vi "Build dotNET Product List.vi"(8 "error in (no error)":errorcluster, 11 "Bundle Builder in":refnum<class "Bundle Builder.lvclass">) -> (0 "error out":errorcluster, 2 "Product List":refnum<k24>[](array[refnum]), 3 "Bundle Builder out":refnum<class "Bundle Builder.lvclass">)   [LabVIEW 2020, in "Bundle Builder.lvclass"]
uses:
  Bundle Builder.lvclass
  C:/Users/chihong/Documents/Repos/StsCustomBundleBuilder/Code/StsCustomBundleBuilder/StsCustomBundleBuilderLib/StsCustomBundleBuilderLib.dll
  StsCustomBundleBuilderLib/StsCustomBundleBuilderLib.dll
  Bundle Builder.lvclass/Bundle Builder.ctl
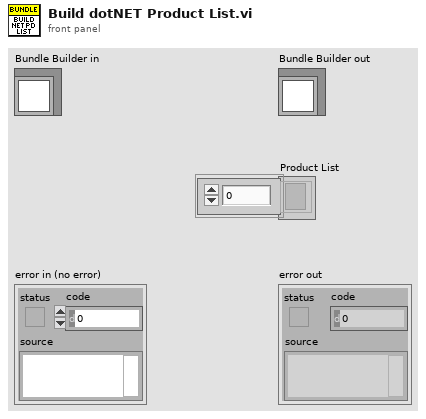
[diagram p1: front panel]
types:
  T1 = cluster{"Display Name":string, "Type":enum16{"NI Installer", "Custom Installer"}, "Install Commands":cluster{"Path":string, "Parameters":string, "Successful Exit Codes":string, "Log Command":cluster{"Flag":string, "File Name":string}}[], "Uninstall Commands":cluster{"Path":string, "Parameters":string, "Successful Exit Codes":string, "Log Command":cluster{"Flag":string, "File Name":string}}[]}[]
  T2 = cluster{"Path":string, "Parameters":string, "Successful Exit Codes":string, "Log Command":cluster{"Flag":string, "File Name":string}}[]
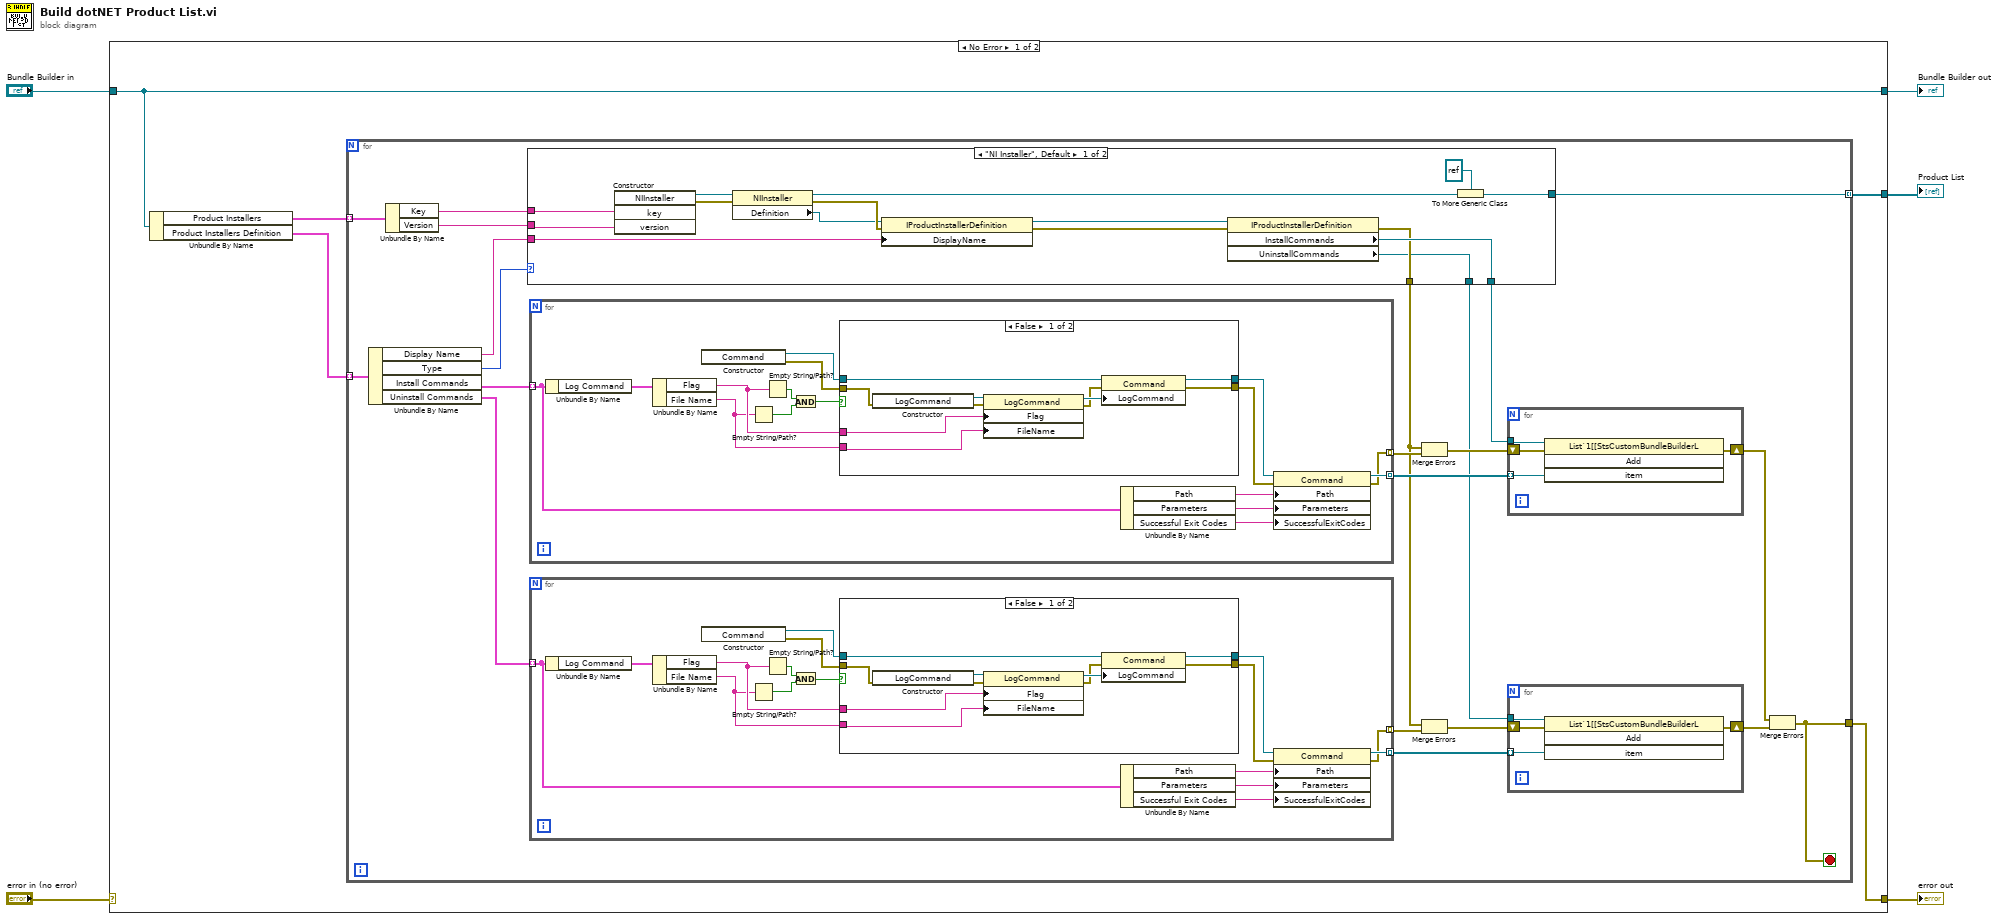
[diagram p0: block diagram]
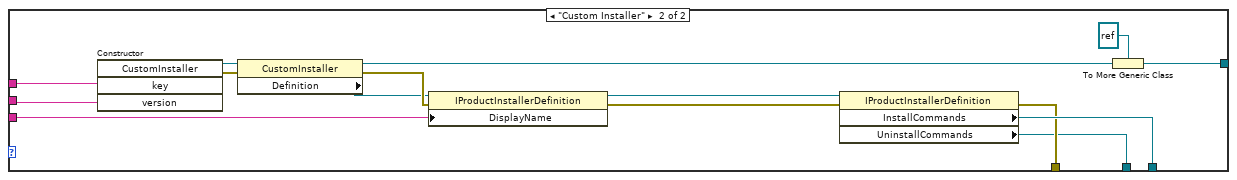
[diagram p3: hidden frame]
diagram:
  n1 = case shown="No Error" "error in (no error)" {
    selector: "error in (no error)" -> [_ w127]
    tunnel: [w7 w127] -> w4
    tunnel: [w8 w126] -> w2
    tunnel: "Bundle Builder in" -> [w8 w126]
    tunnel: [w6 _] -> w1
    frame No Error {
      n2 = Unbundle By Name(w8) -> ("Product Installers"=w10:cluster{"Key":string, "Version":string}[], "Product Installers Definition"=w9:T1)
      n3 = for {
        tunnel: w10 -> [w28] mode=indexing
        tunnel: w9 -> [w31] mode=indexing
        tunnel: [w12] -> w7
        tunnel: [w11] -> w6 mode=indexing
        stop <- w12 stop-if-true
        n4 = Unbundle By Name(w31) -> ("Display Name"=w27:string, "Type"=w29:enum16{"NI Installer", "Custom Installer"}, "Install Commands"=w30:T2, "Uninstall Commands"=w17:T2)
        n5 = Unbundle By Name(w28) -> ("Key"=w25:string, "Version"=w26:string)
        n6 = case shown="\"NI Installer\", Default" w29 {
          tunnel: w27 -> [w81 w96]
          tunnel: w26 -> [w74 w89]
          tunnel: w25 -> [w75 w90]
          tunnel: [w79 w94] -> w24
          tunnel: [w77 w92] -> w16
          tunnel: [w76 w91] -> w15
          tunnel: [w68 w83] -> w11
          frame "NI Installer", Default {
            n7 = constructor class="NIInstaller"("key"=w75, "version"=w74) -> (reference out=w72:refnum<k24>, error out=w82:errorcluster)  [unwired: 3 in, 3 out]
            n8 = property class="NIInstaller"(reference=w72, error in=w82) -> (reference out=w69:refnum<k24>, error out=w73:errorcluster, "Definition"=w71:refnum<k24>)
            n9 = property class="IProductInstallerDefinition"(reference=w71, error in=w73, "DisplayName"=w81) -> (reference out=w80:refnum<k24>, error out=w78:errorcluster)
            n10 = property class="IProductInstallerDefinition"(reference=w80, error in=w78) -> (error out=w77:errorcluster, "InstallCommands"=w79:refnum<k24>, "UninstallCommands"=w76:refnum<k24>)  [unwired: 1 out]
            n11 = To More Generic Class(target class=refnum<k24> refnum ("new reference"), reference=w69) -> (generic class reference=w68:refnum<k24>)
          }
          frame "Custom Installer" {
            n12 = constructor class="CustomInstaller"("key"=w90, "version"=w89) -> (reference out=w87:refnum<k24>, error out=w97:errorcluster)  [unwired: 3 in, 3 out]
            n13 = property class="CustomInstaller"(reference=w87, error in=w97) -> (reference out=w84:refnum<k24>, error out=w88:errorcluster, "Definition"=w86:refnum<k24>)
            n14 = property class="IProductInstallerDefinition"(reference=w86, error in=w88, "DisplayName"=w96) -> (reference out=w95:refnum<k24>, error out=w93:errorcluster)
            n15 = property class="IProductInstallerDefinition"(reference=w95, error in=w93) -> (error out=w92:errorcluster, "InstallCommands"=w94:refnum<k24>, "UninstallCommands"=w91:refnum<k24>)  [unwired: 1 out]
            n16 = To More Generic Class(target class=refnum<k24> refnum ("new reference"), reference=w84) -> (generic class reference=w83:refnum<k24>)
          }
        }
        n17 = for {
          tunnel: w30 -> [w106] mode=indexing
          tunnel: [w101] -> w21 mode=indexing
          tunnel: [w98] -> w23 mode=indexing
          n18 = Unbundle By Name(w106) -> ("Log Command"=w113:cluster{"Flag":string, "File Name":string})
          n19 = Unbundle By Name(w113) -> ("Flag"=w108:string, "File Name"=w107:string)
          n20 = constructor class="Command"() -> (reference out=w109:refnum<k24>, error out=w100:errorcluster)  [unwired: 3 in, 1 out]
          n21 = Empty String/Path?(string/path=w107) -> (empty?=w111:bool)
          n22 = Empty String/Path?(string/path=w108) -> (empty?=w112:bool)
          n23 = And(x=w112, y=w111) -> (x .and. y?=w110:bool)
          n24 = case shown="False" w110 {
            tunnel: w109 -> [w120 w125]
            tunnel: w108 -> [w122 _]
            tunnel: w107 -> [w121 _]
            tunnel: [w118 w125] -> w105
            tunnel: w100 -> [w117 w124]
            tunnel: [w114 w124] -> w99
            frame False {
              n25 = constructor class="LogCommand"(error in=w117) -> (reference out=w123:refnum<k24>, error out=w116:errorcluster)  [unwired: 2 in, 1 out]
              n26 = property class="LogCommand"(reference=w123, error in=w116, "Flag"=w122, "FileName"=w121) -> (reference out=w119:refnum<k24>, error out=w115:errorcluster)
              n27 = property class="Command"(reference=w120, error in=w115, "LogCommand"=w119) -> (reference out=w118:refnum<k24>, error out=w114:errorcluster)
            }
            frame True {
              # "Empty Log Command. \nNo need create."
            }
          }
          n28 = Unbundle By Name(w106) -> ("Path"=w104:string, "Parameters"=w103:string, "Successful Exit Codes"=w102:string)
          n29 = property class="Command"(reference=w105, error in=w99, "Path"=w104, "Parameters"=w103, "SuccessfulExitCodes"=w102) -> (reference out=w101:refnum<k24>, error out=w98:errorcluster)
        }
        n30 = for {
          tunnel: w17 -> [w44] mode=indexing
          tunnel: [w39] -> w20 mode=indexing
          tunnel: [w36] -> w18 mode=indexing
          n31 = Unbundle By Name(w44) -> ("Log Command"=w51:cluster{"Flag":string, "File Name":string})
          n32 = Unbundle By Name(w51) -> ("Flag"=w46:string, "File Name"=w45:string)
          n33 = constructor class="Command"() -> (reference out=w47:refnum<k24>, error out=w38:errorcluster)  [unwired: 3 in, 1 out]
          n34 = Empty String/Path?(string/path=w45) -> (empty?=w49:bool)
          n35 = Empty String/Path?(string/path=w46) -> (empty?=w50:bool)
          n36 = And(x=w50, y=w49) -> (x .and. y?=w48:bool)
          n37 = case shown="False" w48 {
            tunnel: w47 -> [w58 w63]
            tunnel: w46 -> [w60 _]
            tunnel: w45 -> [w59 _]
            tunnel: [w56 w63] -> w43
            tunnel: w38 -> [w55 w62]
            tunnel: [w52 w62] -> w37
            frame False {
              n38 = constructor class="LogCommand"(error in=w55) -> (reference out=w61:refnum<k24>, error out=w54:errorcluster)  [unwired: 2 in, 1 out]
              n39 = property class="LogCommand"(reference=w61, error in=w54, "Flag"=w60, "FileName"=w59) -> (reference out=w57:refnum<k24>, error out=w53:errorcluster)
              n40 = property class="Command"(reference=w58, error in=w53, "LogCommand"=w57) -> (reference out=w56:refnum<k24>, error out=w52:errorcluster)
            }
            frame True {
              # "Empty Log Command. \nNo need create."
            }
          }
          n41 = Unbundle By Name(w44) -> ("Path"=w42:string, "Parameters"=w41:string, "Successful Exit Codes"=w40:string)
          n42 = property class="Command"(reference=w43, error in=w37, "Path"=w42, "Parameters"=w41, "SuccessfulExitCodes"=w40) -> (reference out=w39:refnum<k24>, error out=w36:errorcluster)
        }
        n43 = Merge Errors(w16, w23) -> (w22:errorcluster)
        n44 = Merge Errors(w16, w18) -> (w19:errorcluster)
        n45 = for {
          tunnel: w24 -> [w67]
          shift-right: [w64] -> w13
          shift-left: w22 -> [w66]
          tunnel: w21 -> [w65] mode=indexing
          n46 = invoke class="List`1[[StsCustomBundleBuilderL" method="Add"(reference=w67, error in=w66, "item"=w65) -> (error out=w64:errorcluster)  [unwired: 1 in, 3 out]
        }
        n47 = for {
          tunnel: w15 -> [w35]
          shift-right: [w32] -> w14
          shift-left: w19 -> [w34]
          tunnel: w20 -> [w33] mode=indexing
          n48 = invoke class="List`1[[StsCustomBundleBuilderL" method="Add"(reference=w35, error in=w34, "item"=w33) -> (error out=w32:errorcluster)  [unwired: 1 in, 3 out]
        }
        n49 = Merge Errors(w13, w14) -> (w12:errorcluster)
      }
    }
    frame Error {
    }
  }
  "error out" <- w4
  "Bundle Builder out" <- w2
  "Product List" <- w1
